vi "FTW-TestExecutive-LoadSequence.vi"(0 "FTW Actor Connector In":refnum<class "FTW-ActorConnector.lvclass">, 7 "Script":string, 11 "error in (no error)":errorcluster) -> (4 "FTW Actor Connector":refnum<class "FTW-ActorConnector.lvclass">, 8 "Loaded Sequence":T1[](array[typedef]) {"Elapsed Time" format="%<%H:%M:%S%3u>t"}, 14 "Roundtrip Time":dbl format="%.6f sec", 15 "error out":errorcluster)   [LabVIEW 2015]
uses:
  source/actor/Connector/FTW-ActorConnector.lvclass
  FTW-TestExecutive_Step.ctl
  source/JSON/core/FTW-JSON-Core-EncodingFlags.vi
  source/JSON/FTW-JSON-Parse.vi
  source/Reflection/FTW-Reflection-Type.vi
  source/CodeGen/JSON Deserialize/FTW-JSON-Core-GetFlattenedValue.vi
  source/CodeGen/JSON Deserialize/FTW-JSON-Deserialize.xnode
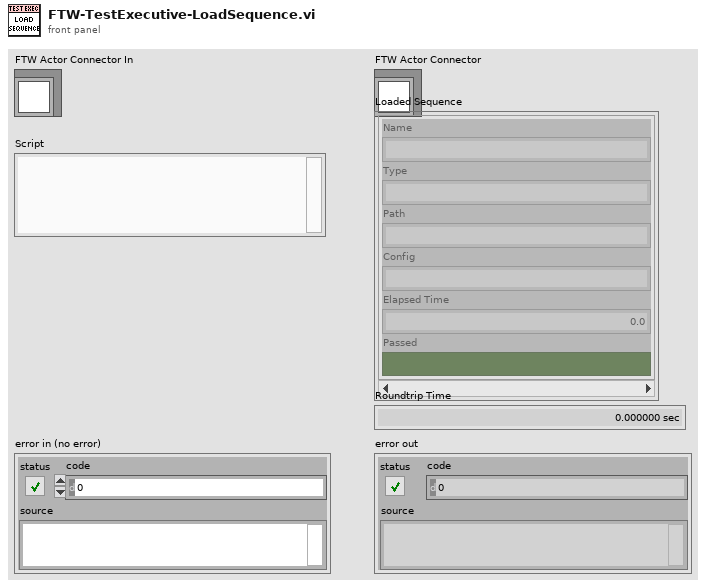
[diagram p1: front panel]
types:
  T1 = typedef "FTW-TestExecutive_Step.ctl" = cluster{"Name":string, "Type":string, "Path":string, "Config":string, "Elapsed Time":dbl, "Passed":bool}
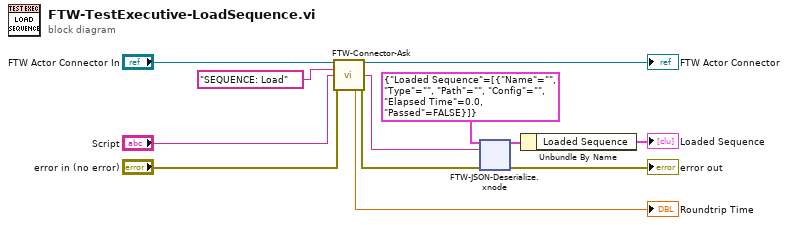
[diagram p0: block diagram]
diagram:
  n1 = call "FTW-Connector-Ask.vi"("FTW Actor Connector"="FTW Actor Connector In", "Request Header"="SEQUENCE: Load", "Request Body"="Script", "error in"="error in (no error)") -> ("FTW Actor Connector out"=→"FTW Actor Connector":refnum<class "FTW-ActorConnector.lvclass">, "Response Body"=w5:string, "Roundtrip Time"=→"Roundtrip Time":dbl, "error out"=w8:errorcluster)  [unwired: 6 in, 2 out]
  n2 = xnode "FTW-JSON-Deserialize.xnode"("Type and Defaults"=cluster{"Loaded Sequence":T1[]} {"Loaded Sequence"=[{"Name"="", "Type"="", "Path"="", "Config"="", "Elapsed Time"=0.0, "Passed"=FALSE}]}, "JSON String"=w5, "error in"=w8) -> ("Values"=w3:cluster{"Loaded Sequence":T1[]}, "error out"=→"error out":errorcluster)
  n3 = Unbundle By Name(w3) -> ("Loaded Sequence"=→"Loaded Sequence":T1[])
